vi "Radial_Deadzone.vi"(0 "Squared":bool, 1 "X":dbl, 2 "Y":dbl, 3 "Band":dbl) -> (4 "Not_Zero":bool, 5 "X_Out":dbl, 6 "Y_Out":dbl)   [LabVIEW 2018]
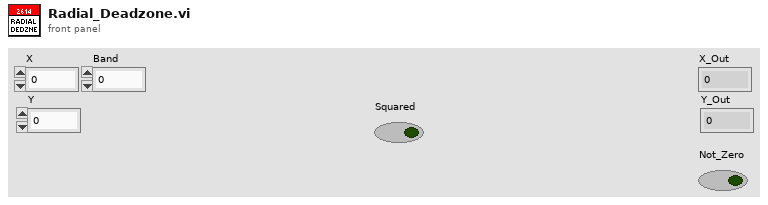
[diagram p1: front panel]
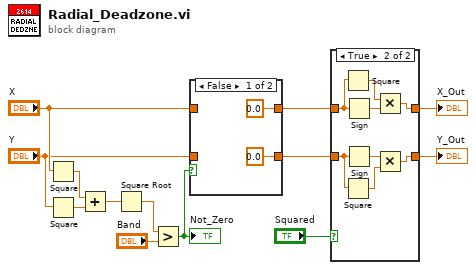
[diagram p0: block diagram]
diagram:
  n1 = Square(x="X") -> (x^2=w12:dbl)
  n2 = Square(x="Y") -> (x^2=w11:dbl)
  n3 = Add(x=w12, y=w11) -> (x+y=w13:dbl)
  n4 = Square Root(x=w13) -> (sqrt(x)=w10:dbl)
  n5 = Greater?(x=w10, y="Band") -> (0:w6:bool)
  "Not_Zero" <- w6
  n6 = case shown="False" w6 {
    tunnel: "X" -> [_ w16]
    tunnel: "Y" -> [_ w17]
    tunnel: [0.0 ("Y") w17] -> w4
    tunnel: [0.0 ("X") w16] -> w2
    frame False {
    }
    frame True {
    }
  }
  n7 = case shown="True" "Squared" {
    tunnel: [w18 w24] -> w5
    tunnel: w4 -> [w18 w22]
    tunnel: [w19 w25] -> w3
    tunnel: w2 -> [w19 w23]
    frame False {
    }
    frame True {
      n8 = Square(x=w23) -> (x^2=w27:dbl)
      n9 = Square(x=w22) -> (x^2=w26:dbl)
      n10 = Sign(1:w23) -> (0:w21:dbl)
      n11 = Sign(1:w22) -> (0:w20:dbl)
      n12 = Multiply(x=w27, y=w21) -> (x*y=w25:dbl)
      n13 = Multiply(x=w20, y=w26) -> (x*y=w24:dbl)
    }
  }
  "X_Out" <- w3
  "Y_Out" <- w5
